vi "Write Motor PID Gains.vi"(8 "error in (no error)":errorcluster, 10 "motor PID gains":T1={"proportional gain (Kc)"=0.25, "integral gain (Kc*Ts/Ti)"=0.3984375, "derivative gain (Kc*Td/Ts)"=0.01171875}, 11 "starter kit host in":refnum<class "NI_Robotics_Starter Kit Host.lvclass">) -> (0 "error out":errorcluster, 3 "starter kit host out":refnum<class "NI_Robotics_Starter Kit Host.lvclass">)   [LabVIEW 2017, in "NI_Robotics_Starter Kit Host.lvclass"]
uses:
  <vilib>/robotics/Starter Kit/Host Interface/NI_Robotics_Starter Kit Host.lvclass
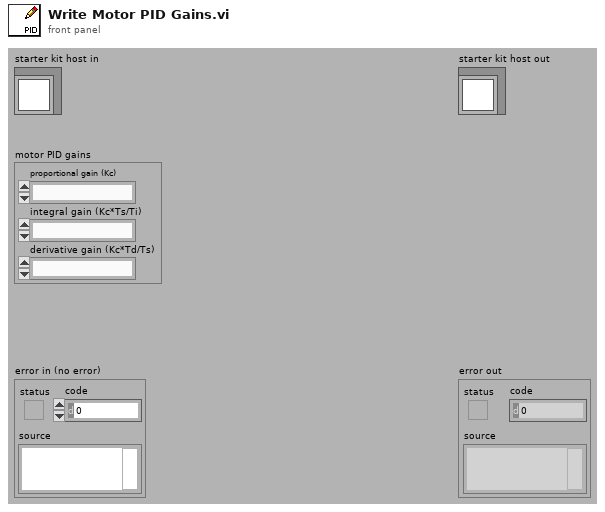
[diagram p1: front panel]
types:
  T1 = cluster{"proportional gain (Kc)":fxp<+/-,16,8>, "integral gain (Kc*Ts/Ti)":fxp<+/-,16,8>, "derivative gain (Kc*Td/Ts)":fxp<+/-,16,8>}
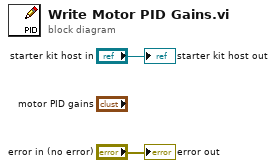
[diagram p0: block diagram]
diagram:
  "error out" <- "error in (no error)"
  "starter kit host out" <- "starter kit host in"
